vi "Read activeChannel.vi"(8 "error in (no error)":errorcluster, 11 "HexapodPI in":refnum<class "HexapodPI.lvclass">) -> (0 "error out":errorcluster, 2 "active axis":T1, 3 "HexapodPI out":refnum<class "HexapodPI.lvclass">)   [LabVIEW 2020, in "HexapodPI.lvclass"]
uses:
  HexapodPI.lvclass
  subvis/activeChannel.ctl
  HexapodPI.lvclass/HexapodPI.ctl
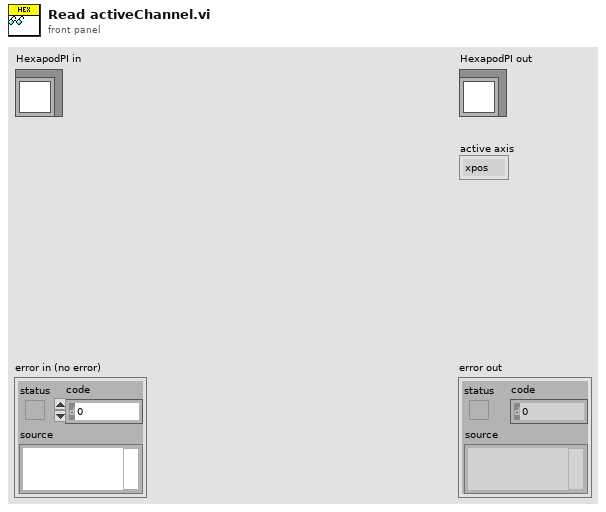
[diagram p1: front panel]
types:
  T1 = typedef "activeChannel.ctl" = enum16{"xpos", "ypos", "zpos", "uangle", "vangle", "wangle", "n/a", "off"}
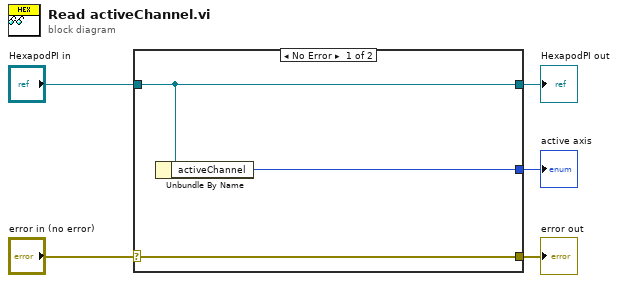
[diagram p0: block diagram]
diagram:
  n1 = case shown="No Error" "error in (no error)" {
    selector: "error in (no error)" -> [w8 w9]
    tunnel: [w8 w9] -> w4
    tunnel: [w7 w10] -> w2
    tunnel: "HexapodPI in" -> [w7 w10]
    tunnel: [w6 _] -> w1
    frame No Error {
      n2 = Unbundle By Name(w7) -> ("activeChannel"=w6:T1)
    }
    frame Error {
    }
  }
  "error out" <- w4
  "HexapodPI out" <- w2
  "active axis" <- w1
